vi "Parse server response.vi"(8 "error in (no error)":errorcluster, 10 "expected response":T1 items=["detailed response", "stop", "ping"], 11 "server response in":string) -> (0 "error out":errorcluster, 1 "detailed error info":T2, 2 "JSON out":string, 3 "binary data":u8[](array[numeric]), 4 "Protocoll version":u8, 5 "return code":u8, 6 "optional header":u8[](array[numeric]), 7 "jl stack trace":bool)   [LabVIEW 2018, in "LV2Julia_core.lvlib"]
uses:
  LV2Julia_core.lvlib
  detailed error info.ctl
  StackFrame.ctl
  expected server response.ctl
  prot version global.vi
  <vilib>/Utility/error.llb/Error Cluster From Error Code.vi
  <vilib>/ErrorRing/Error Ring.xnode
panel:
  out "response type as expected":bool
  out "binary data length":u32
  out "optional header length":u32
  out "unsigned byte array":u8[](array[numeric])
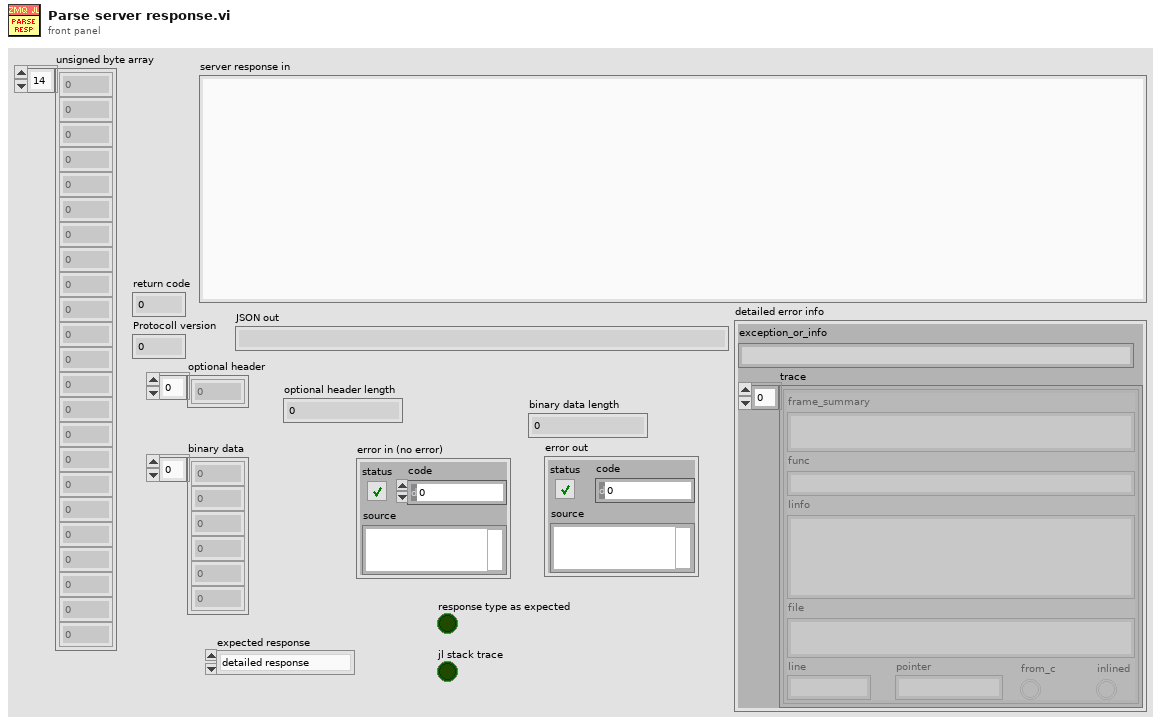
[diagram p1: front panel]
types:
  T1 = typedef "LV2Julia_core.lvlib/expected server response.ctl" = u16
  T2 = typedef "LV2Julia_core.lvlib/detailed error info.ctl" = cluster{"exception_or_info":string, "trace":T3[]}
  T3 = typedef "LV2Julia_core.lvlib/StackFrame.ctl" = cluster{"frame_summary":string, "func":string, "linfo":string, "file":string, "line":i32, "pointer":u64, "from_c":bool, "inlined":bool}
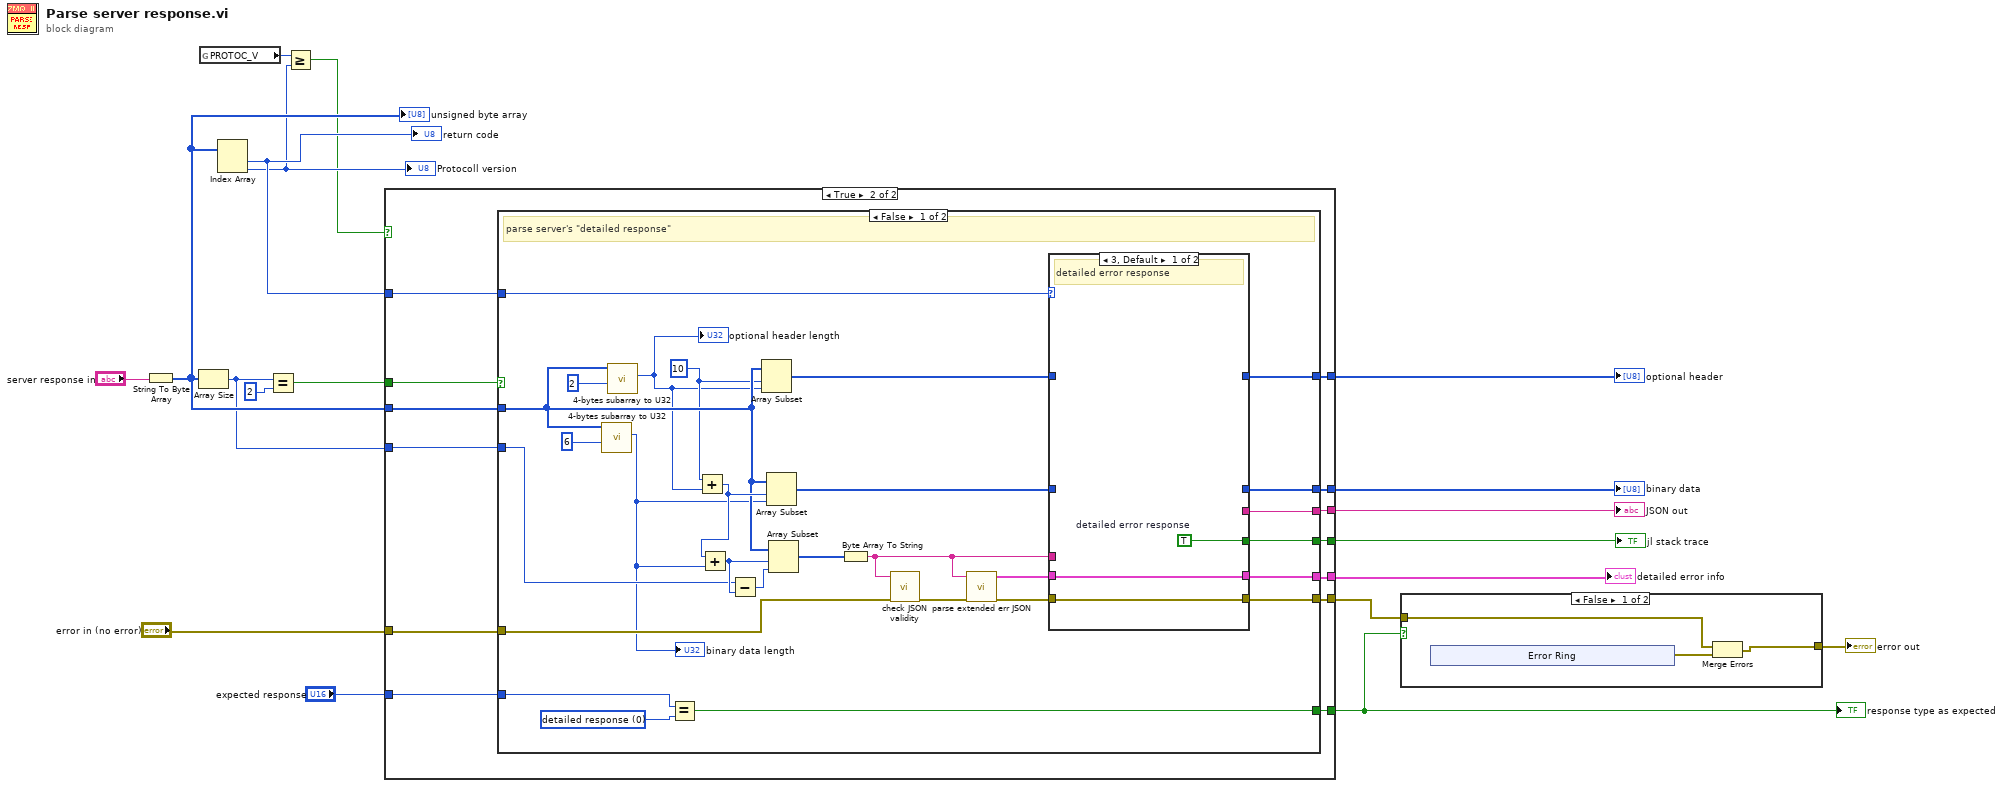
[diagram p0: block diagram]
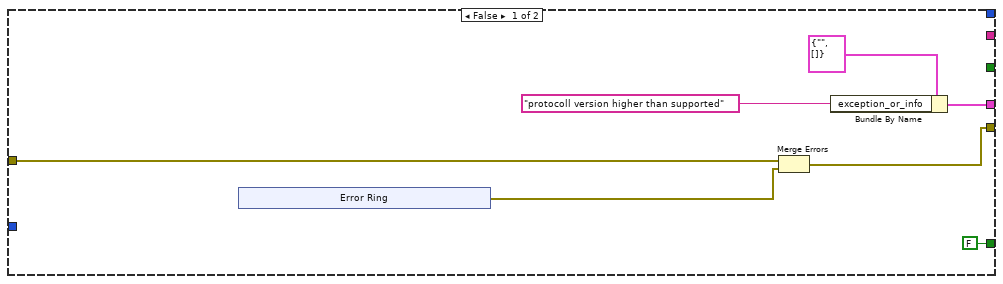
[diagram p3: hidden frame]
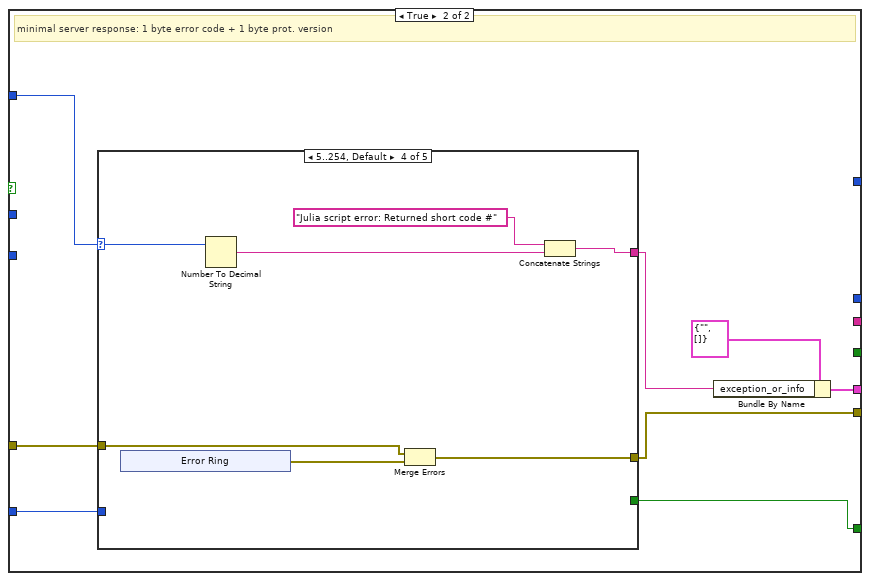
[diagram p5: hidden frame]
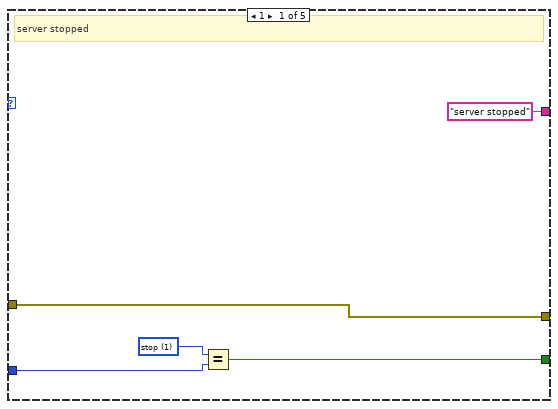
[diagram p6: hidden frame]
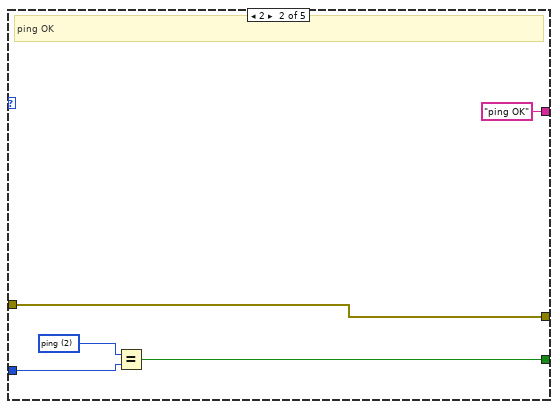
[diagram p7: hidden frame]
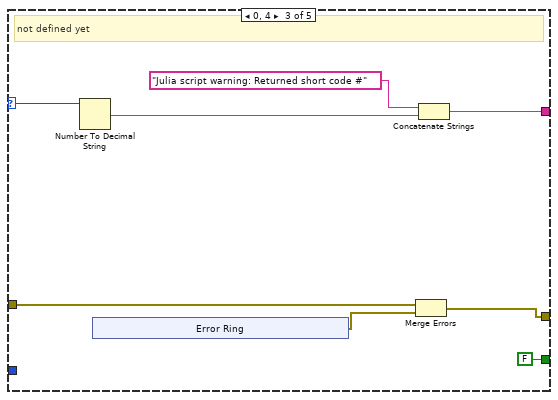
[diagram p8: hidden frame]
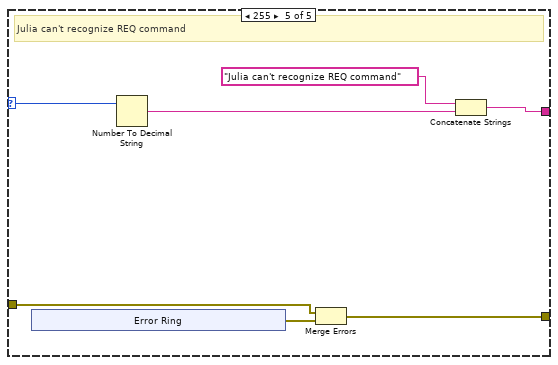
[diagram p9: hidden frame]
diagram:
  n1 = String To Byte Array(string="server response in") -> (unsigned byte array=w14:u8[])
  "unsigned byte array" <- w14
  n2 = Array Size(array=w14) -> (size(s)=w13:i32)
  n3 = global read "prot version global.vi" "PROTOC_V"() -> (w8:u8)
  n4 = Index Array(array=w14) -> (element #1=w10:u8, element #2=w7:u8)  [unwired: 2 in]
  "return code" <- w10
  "Protocoll version" <- w7
  n5 = Equal?(x=w13, y=2) -> (x = y?=w11:bool)
  n6 = Greater Or Equal?(x=w8, y=w7) -> (x >= y?=w6:bool)
  n7 = case shown="True" w6 {
    tunnel: [_ w44] -> w18
    tunnel: [_ w43] -> w17
    tunnel: "error in (no error)" -> [w23 w42]
    tunnel: [_ w41] -> w15
    tunnel: [w21 w40] -> w3
    tunnel: w14 -> [_ w39]
    tunnel: w13 -> [_ w38]
    tunnel: w11 -> [_ w37]
    tunnel: w10 -> [_ w36]
    tunnel: [w25 w35] -> w9
    tunnel: "expected response" -> [_ w34]
    tunnel: [FALSE w33] -> w4
    tunnel: [_ w32] -> w1
    frame False {
      n8 = xnode "Error Ring"() -> ("error out"=w22:errorcluster)
      n9 = Merge Errors(w23, w22) -> (w21:errorcluster)
      n10 = Bundle By Name(cluster=T2 {"exception_or_info"="", "trace"=[]} ("detailed error info"), "exception_or_info"="protocoll version higher than supported") -> (w25:T2)
    }
    frame True {
      n11 = case shown="False" w37 {
        tunnel: [w54 _] -> w44
        tunnel: [w49 w83] -> w35
        tunnel: [w53 _] -> w43
        tunnel: w39 -> [w62 _]
        tunnel: w42 -> [w64 w87]
        tunnel: [w52 _] -> w41
        tunnel: [w51 w88] -> w40
        tunnel: w38 -> [w63 _]
        tunnel: w36 -> [w50 w86]
        tunnel: w34 -> [w47 w82]
        tunnel: [w46 w81] -> w33
        tunnel: [w45 _] -> w32
        frame False {
          w48 = T1 0 items=["detailed response", "stop", "ping"] ("expected response")
          w61 = 10 ("index")
          # "parse server's \"detailed response\""
          n12 = call "4-bytes subarray to U32.vi"("offset"=6 ("index"), "unsigned byte array"=w62) -> ("U32 Out"=w60:u32)  [unwired: 8 in, 1 out]
          "binary data length" <- w60
          n13 = call "4-bytes subarray to U32.vi"("offset"=2 ("index"), "unsigned byte array"=w62) -> ("U32 Out"=w59:u32)  [unwired: 8 in, 1 out]
          "optional header length" <- w59
          n14 = Equal?(x=w47, y=w48) -> (x = y?=w46:bool)
          n15 = Add(x=w61, y=w59) -> (x+y=w68:u32)
          n16 = Add(x=w68, y=w60) -> (x+y=w67:u32)
          n17 = Subtract(x=w63, y=w67) -> (x-y=w66:u32)
          n18 = Array Subset(array=w62, index=w61, length=w59) -> (w70:u8[])
          n19 = Array Subset(array=w62, index=w68, length=w60) -> (w69:u8[])
          n20 = Array Subset(array=w62, index=w67, length=w66) -> (w65:u8[])
          n21 = Byte Array To String(unsigned byte array=w65) -> (string=w58:string)
          n22 = call "check JSON validity.vi"("error in (no error)"=w64, "JSON string in"=w58) -> ("error out"=w57:errorcluster)  [unwired: 8 in, 1 out]
          n23 = call "parse extended err JSON.vi"("error in (no error)"=w57, "JSON string in"=w58) -> ("error out"=w56:errorcluster, "stack trace"=w55:T2)  [unwired: 7 in, 1 out]
          n24 = case shown="3, Default" w50 {
            tunnel: w70 -> [_ w80]
            tunnel: w69 -> [_ w79]
            tunnel: w58 -> [_ w78]
            tunnel: w56 -> [w75 w77]
            tunnel: w55 -> [w74 w76]
            tunnel: [_ w80] -> w54
            tunnel: [_ w79] -> w53
            tunnel: [_ w78] -> w52
            tunnel: [w74 w76] -> w49
            tunnel: [w75 w77] -> w51
            tunnel: [w73 _] -> w45
            frame 3, Default {
              w73 = TRUE  # detailed error response
              # "detailed error response"
            }
            frame 0 {
              # "normal detailed response"
            }
          }
        }
        frame True {
          # "minimal server response: 1 byte error code + 1 byte prot. version"
          n25 = case shown="5..254, Default" w86 {
            selector: w86 -> [_ _ w101 w111 w123]
            tunnel: [w93 w98 w105 w113 w125] -> w88
            tunnel: w87 -> [w93 w98 w106 w112 w124]
            tunnel: ["server stopped" "ping OK" w100 w109 w121] -> w84
            tunnel: w82 -> [w90 w95 _ _ _]
            tunnel: [w89 w94 FALSE _ _] -> w81
            frame 1 {
              w91 = T1 1 items=["detailed response", "stop", "ping"] ("expected response")
              # "server stopped"
              n26 = Equal?(x=w91, y=w90) -> (x = y?=w89:bool)
            }
            frame 2 {
              w96 = T1 2 items=["detailed response", "stop", "ping"] ("expected response")
              # "ping OK"
              n27 = Equal?(x=w96, y=w95) -> (x = y?=w94:bool)
            }
            frame 0, 4 {
              # "not defined yet"
              n28 = Number To Decimal String(number=w101) -> (decimal integer string=w103:string)  [unwired: 1 in]
              n29 = xnode "Error Ring"() -> ("error out"=w104:errorcluster)
              n30 = Merge Errors(w106, w104) -> (w105:errorcluster)
              n31 = Concatenate Strings("Julia script warning: Returned short code #" ("string"), w103) -> (w100:string)
            }
            frame 5..254, Default {
              n32 = xnode "Error Ring"() -> ("error out"=w114:errorcluster)
              n33 = Number To Decimal String(number=w111) -> (decimal integer string=w110:string)  [unwired: 1 in]
              n34 = Merge Errors(w112, w114) -> (w113:errorcluster)
              n35 = Concatenate Strings("Julia script error: Returned short code #" ("string"), w110) -> (w109:string)
            }
            frame 255 {
              # "Julia can't recognize REQ command"
              n36 = xnode "Error Ring"() -> ("error out"=w126:errorcluster)
              n37 = Number To Decimal String(number=w123) -> (decimal integer string=w122:string)  [unwired: 1 in]
              n38 = Merge Errors(w124, w126) -> (w125:errorcluster)
              n39 = Concatenate Strings("Julia can't recognize REQ command" ("string"), w122) -> (w121:string)
            }
          }
          n40 = Bundle By Name(cluster=T2 {"exception_or_info"="", "trace"=[]} ("detailed error info"), "exception_or_info"=w84) -> (w83:T2)
        }
      }
    }
  }
  "optional header" <- w18
  "binary data" <- w17
  "JSON out" <- w15
  "detailed error info" <- w9
  "response type as expected" <- w4
  "jl stack trace" <- w1
  n41 = case shown="False" w4 {
    tunnel: w3 -> [w133 w140]
    tunnel: [w132 w140] -> w2
    frame False {
      n42 = xnode "Error Ring"() -> ("error out"=w134:errorcluster)
      n43 = Merge Errors(w133, w134) -> (w132:errorcluster)
    }
    frame True {
    }
  }
  "error out" <- w2
